vi "Assign Pixel to Wing Sector (Host)Test.vi"(6 "Pixel Intensity In":u8, 7 "Right Wing?":bool, 8 "Sector Parameters":T1, 9 "Pixel Y":u16, 10 "Pixel X":u16) -> (0 "Pixel Y Out":u16, 1 "Pixel Intensity Out":u8, 2 "sector #":u8, 3 "output valid":bool, 4 "Pixel X Out":u16)   [LabVIEW 2013]
uses:
  <vilib>/rvi/FXPMathLib/FxpRectToPolar/subVIs/nifxpmath_RectToPolar_SimConfig.ctl
  <vilib>/rvi/FXPMathLib/FxpDiv/subVIs/nifxpmath_Div_SimConfig.ctl
  <vilib>/rvi/FXPMathLib/FxpRectToPolar/simVIs/DllFxpRectToPolarTemp_sub.vi
  <vilib>/rvi/FXPMathLib/FxpDiv/simVIs/DllFxpDivTemp_sub.vi
  <vilib>/rvi/FXPMathLib/FxpSub/XNode/nifxpmath_Sub.xnode
  <vilib>/rvi/FXPMathLib/FxpRectToPolar/XNode/nifxpmath_RectToPolar.xnode
  <vilib>/rvi/FXPMathLib/FxpAdd/XNode/nifxpmath_Add.xnode
  <vilib>/rvi/FXPMathLib/FxpDiv/XNode/nifxpmath_Div.xnode
  <vilib>/rvi/FXPMathLib/sim/FxpSim.dll
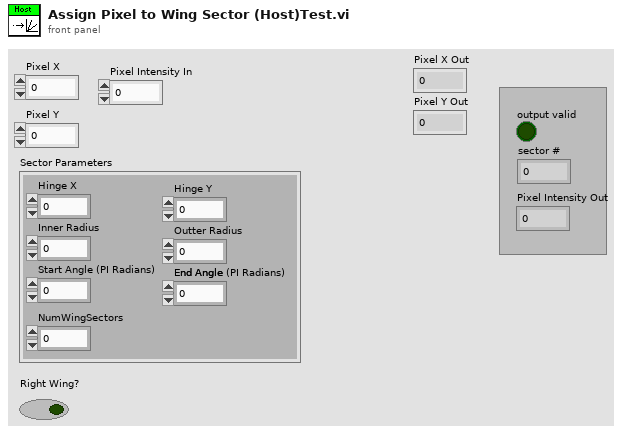
[diagram p1: front panel]
types:
  T1 = cluster{"Start Angle":fxp<+/-,17,2>, "End Angle":fxp<+,17,3>, "Inner Radius":u16, "Outter Radius":u16, "Hinge X":u16, "Hinge Y":u16, "NumWingSectors":u8}
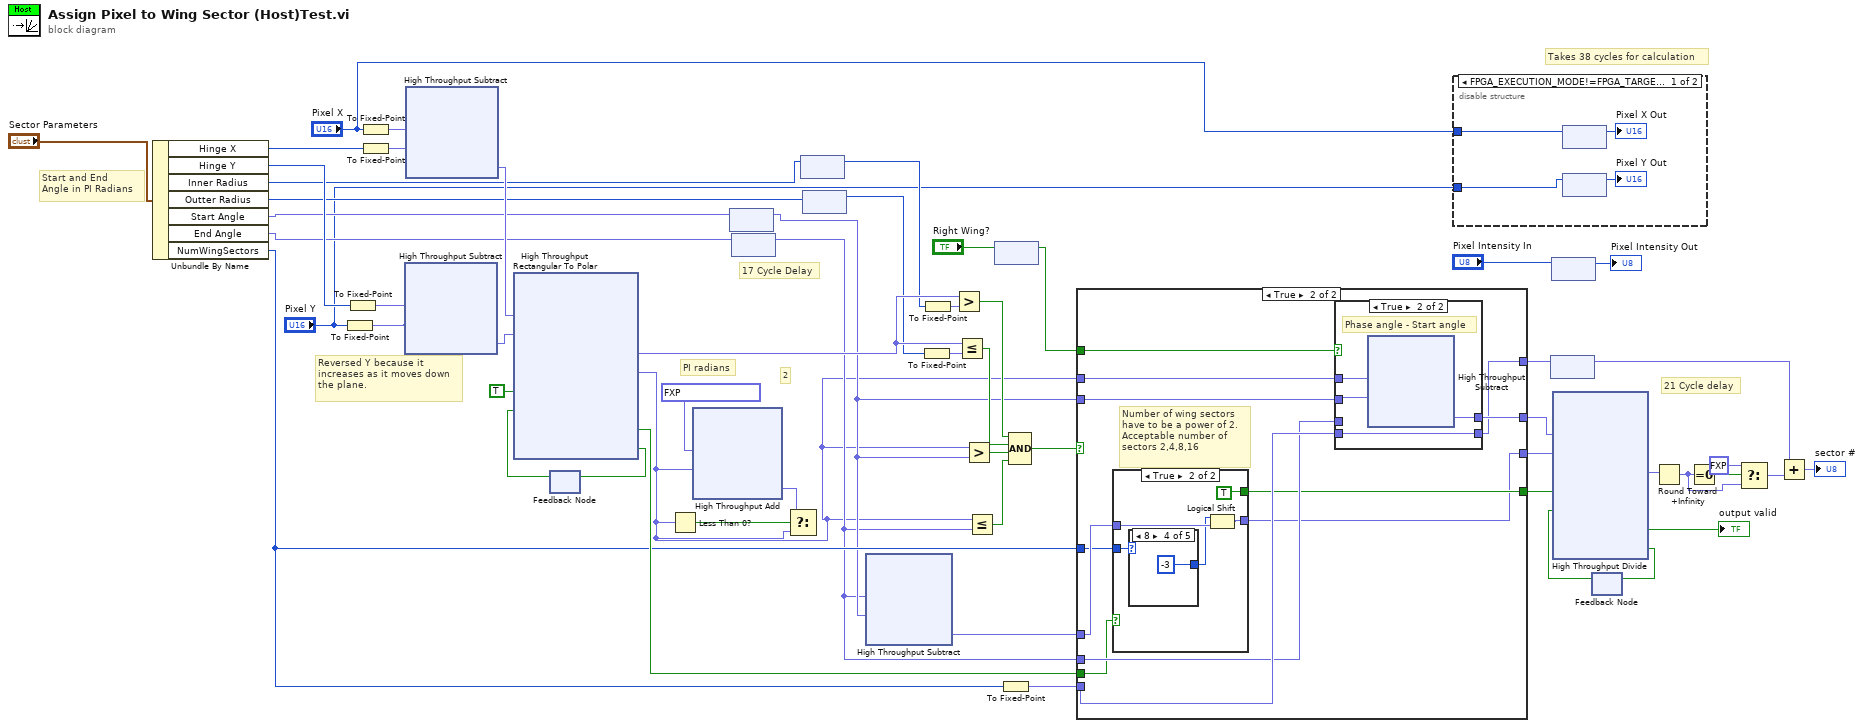
[diagram p0: block diagram]
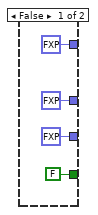
[diagram p3: hidden frame]
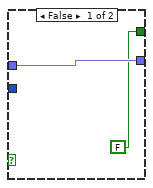
[diagram p4: hidden frame]
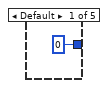
[diagram p5: hidden frame]
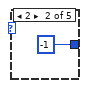
[diagram p6: hidden frame]
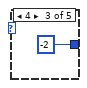
[diagram p7: hidden frame]
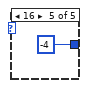
[diagram p8: hidden frame]
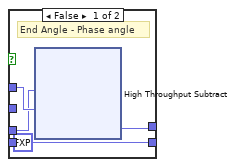
[diagram p9: hidden frame]
diagram:
  # "Takes 38 cycles for calculation"
  # "17 Cycle Delay"
  # "Reversed Y because it\nincreases as it moves down\nthe plane."
  # "PI radians"
  # "21 Cycle delay"
  # "Start and End\nAngle in PI Radians"
  # "2"
  n1 = Unbundle By Name("Sector Parameters") -> ("Hinge X"=w22:u16, "Hinge Y"=w42:u16, "Inner Radius"=w16:u16, "Outter Radius"=w14:u16, "Start Angle"=w12:fxp<+/-,17,2>, "End Angle"=w10:fxp<+,17,3>, "NumWingSectors"=w25:u8)
  n2 = To Fixed-Point(number="Pixel Y") -> (fixed-point=w30:fxp<+,11,11>)  [unwired: 1 in]
  n3 = To Fixed-Point(number=w42) -> (fixed-point=w31:fxp<+,11,11>)  [unwired: 1 in]
  n4 = To Fixed-Point(number="Pixel X") -> (fixed-point=w29:fxp<+,11,11>)  [unwired: 1 in]
  n5 = To Fixed-Point(number=w22) -> (fixed-point=w28:fxp<+,11,11>)  [unwired: 1 in]
  n6 = xnode "High Throughput Subtract"("x"=w31, "y"=w30) -> ("x-y"=w40:fxp<+/-,12,12>)
  n7 = xnode "High Throughput Subtract"("x"=w29, "y"=w28) -> ("x-y"=w39:fxp<+/-,12,12>)
  n8 = feedback #1() -> (w47:bool)  [unwired: 1 in]
  n9 = xnode "High Throughput Rectangular To Polar"("x"=w39, "y"=w40, "input valid"=TRUE, "ready for output (T)"=w47) -> ("magnitude"=w55:fxp<+,12,12>, "phase (pi)"=w1:fxp<+/-,16,2>, "output valid"=w26:bool, "ready for input"=w48:bool)
  n10 = feedback-in #1(w48) -> ()
  n11 = Less Than 0?(x=w1) -> (x < 0?=w52:bool)
  n12 = xnode ("High Throughput Add")("x"=fxp<+/-,16,2> 1.99993896484375 ("y"), "y"=w1) -> ("x+y"=w51:fxp<+/-,17,3>)
  n13 = feedback #2() -> (w11:fxp<+/-,17,2>)  [unwired: 1 in]
  n14 = feedback-in #2(w12) -> ()
  n15 = feedback #3() -> (w9:fxp<+,17,3>)  [unwired: 1 in]
  n16 = feedback-in #3(w10) -> ()
  n17 = Select(t=w51, s=w52, f=w1) -> ()  [unwired: 1 out]
  n18 = feedback #4() -> (w15:u16)  [unwired: 1 in]
  n19 = feedback-in #4(w16) -> ()
  n20 = feedback #5() -> (w13:u16)  [unwired: 1 in]
  n21 = feedback-in #5(w14) -> ()
  n22 = xnode ("High Throughput Subtract")("x"=w9, "y"=w11) -> ("x-y"=w27:fxp<+/-,17,6>)
  n23 = To Fixed-Point(number=w13) -> (fixed-point=w54:fxp<+,16,16>)  [unwired: 1 in]
  n24 = To Fixed-Point(number=w15) -> (fixed-point=w56:fxp<+,16,16>)  [unwired: 1 in]
  n25 = Greater?(x=w55, y=w56) -> (0:w46:bool)
  n26 = Less Or Equal?(x=w55, y=w54) -> (x <= y?=w45:bool)
  n27 = Greater?(x=w1, y=w11) -> (0:w44:bool)
  n28 = Less Or Equal?(x=w1, y=w9) -> (x <= y?=w43:bool)
  n29 = feedback #6() -> (w20:bool)  [unwired: 1 in]
  n30 = feedback-in #6("Right Wing?") -> ()
  n31 = To Fixed-Point(number=w25) -> (fixed-point=w41:fxp<+,8,8>)  [unwired: 1 in]
  n32 = Compound Arithmetic op=AND(w46, w45, w44, w43) -> (w53:bool)
  n33 = case shown="True" w53 {
    tunnel: w1 -> [_ w72]
    tunnel: w11 -> [_ w71]
    tunnel: [fxp<+/-,17,6> 0.0 ("x-y") w62] -> w35
    tunnel: w9 -> [_ w69]
    tunnel: w41 -> [_ w70]
    tunnel: [fxp<+/-,19,5> 0.0 ("x-y") w68] -> w36
    tunnel: [FALSE ("output valid") w63] -> w34
    tunnel: [fxp<+,8,8> 0.0 w67] -> w32
    tunnel: w27 -> [_ w66]
    tunnel: w26 -> [_ w65]
    tunnel: w25 -> [_ w64]
    tunnel: w20 -> [_ w61]
    frame False {
    }
    frame True {
      # "Number of wing sectors\nhave to be a power of 2.\nAcceptable number of\nsectors 2,4,8,16"
      n34 = case shown="True" w65 {
        tunnel: w64 -> [_ w79]
        tunnel: w66 -> [w74 w78]
        tunnel: [w74 w76] -> w62
        tunnel: [FALSE ("output valid") TRUE ("output valid")] -> w63
        frame False {
        }
        frame True {
          n35 = case shown="8" w79 {
            tunnel: [i16 0 ("y") i16 -1 ("y") i16 -2 ("y") i16 -3 ("y") i16 -4 ("y")] -> w77
            frame Default {
            }
            frame 2 {
            }
            frame 4 {
            }
            frame 8 {
            }
            frame 16 {
            }
          }
          n36 = Logical Shift(y=w77, x=w78) -> (x << y=w76:fxp<+/-,17,6>)
        }
      }
      n37 = case shown="True" w61 {
        tunnel: w72 -> [w87 w92]
        tunnel: w71 -> [_ w91]
        tunnel: [w88 w90] -> w68
        tunnel: w70 -> [_ w89]
        tunnel: [fxp<+,8,8> 0.0 w89] -> w67
        tunnel: w69 -> [w86 _]
        frame False {
          # "End Angle - Phase angle"
          n38 = xnode "High Throughput Subtract"("x"=w86, "y"=w87) -> ("x-y"=w88:fxp<+/-,19,5>)
        }
        frame True {
          # "Phase angle - Start angle"
          n39 = xnode ("High Throughput Subtract")("x"=w92, "y"=w91) -> ("x-y"=w90:fxp<+/-,18,3>)
        }
      }
    }
  }
  n40 = disable-structure shown="FPGA_EXECUTION_MODE!=FPGA_TARGET" {
    disable-tunnel: "Pixel X" -> [w96 _]
    disable-tunnel: "Pixel Y" -> [w95 _]
    frame condition #0 (active) {
      n41 = feedback #7() -> (→"Pixel X Out":u16)  [unwired: 1 in]
      n42 = feedback-in #7(w96) -> ()
      n43 = feedback #8() -> (→"Pixel Y Out":u16)  [unwired: 1 in]
      n44 = feedback-in #8(w95) -> ()
    }
    frame condition #1 {
    }
  }
  n45 = feedback #9() -> (w6:fxp<+,8,8>)  [unwired: 1 in]
  n46 = feedback-in #9(w32) -> ()
  n47 = feedback #10() -> (→"Pixel Intensity Out":u8)  [unwired: 1 in]
  n48 = feedback-in #10("Pixel Intensity In") -> ()
  n49 = feedback #11() -> (w33:bool)  [unwired: 1 in]
  n50 = xnode "High Throughput Divide"("x"=w36, "y"=w35, "input valid"=w34, "ready for output (T)"=w33) -> ("x/y"=w19:fxp<+/-,20,16>, "output valid"=→"output valid":bool, "ready for input"=w38:bool)
  n51 = feedback-in #11(w38) -> ()
  n52 = Round Toward +Infinity(x=w19) -> (ceil(x): smallest int >= x=w18:fxp<+/-,17,17>)
  n53 = Equal To 0?(x=w18) -> (x = 0?=w5:bool)
  n54 = Select(t=fxp<+/-,17,17> 1.0, s=w5, f=w18) -> (s? t:f=w8:fxp<+/-,17,17>)
  n55 = Add(x=w6, y=w8) -> (x+y=→"sector #":fxp<+/-,17,17>)
